vi "SV TDMS Read Scalar (N Ch).vi"(0 "tdms file":refnum<k34>, 1 "offset (0)":i64, 2 "count (-1: all)":i64=-1, 5 "group name in":string, 7 "channel names in":string[](array[string]), 11 "error in":errorcluster) -> (3 "scale labels":T1(array[cluster]), 4 "tdms file out":refnum<k34>, 6 "group name out":string, 8 "channel names out":string[](array[string]), 10 "values":dbl[][](array[numeric]), 13 "scalar function info":T2={"scalar function type"=10, "scalar function subtype"=19, " x-dimension"=0} {"scalar function type" items=["Speed"=3, "Ratio"=6, "Count"=7, "-"=9, "Level"=10, "-"=19, "None"=98]; "scalar function subtype" items=["Value"=19, "DC"=11, "AC"=12, "RMS^2"=13, "RMS"=14, "Peak"=15, "Peak to peak"=16, "-"=20, "Phase"=33, "-"=90, "None"=98, "Unknown"=99]; "x-dimension" items=["Time (s)"=0, "Frequency-CB (Hz)"=1, "Frequency-CPB (Hz)"=1248, "Frequency-Arbitrary (Hz)"=2357, "Quefrency (s)"=2, "Revolutions (rev)"=3, "Order"=4, "Speed (RPM)"=11, "Speed (rad/s)"=21, "Critical Band"=31, "Critical Band Rate (Bark)"=32, "None"=98, "Index"=65535]}, 14 "end of file":bool, 15 "error out":errorcluster)   [LabVIEW 2017]
doc: "Reads the specified .tdms file and returns data in a format specific to the polymorphic instance selected."
uses:
  <vilib>/addons/_NISVFA/_Shared subVIs/Controls/NI Scalar Function Info.ctl
  <vilib>/addons/_NISVFA/_Shared subVIs/Controls/svc_X-Axis Units.ctl
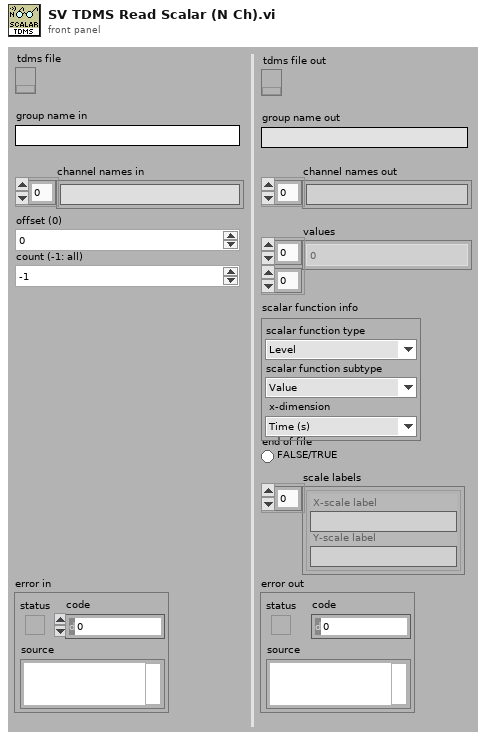
[diagram p1: front panel]
types:
  T1 = cluster{"X-scale label":string, "Y-scale label":string}[]
  T2 = typedef "NI Scalar Function Info.ctl" = cluster{"scalar function type":u16, "scalar function subtype":u16, " x-dimension":T3}
  T3 = typedef "svc_X-Axis Units.ctl" = u16
  T4 = typedef "NI Function Info.ctl" = cluster{"function type":T5, "function subtype":T6, "X-dimension":T3}
  T5 = typedef "NI Function Type.ctl" = u16
  T6 = typedef "NI Function SubType.ctl" = u16
  T7 = cluster{"X-scale label":string, "Y-scale label":string}
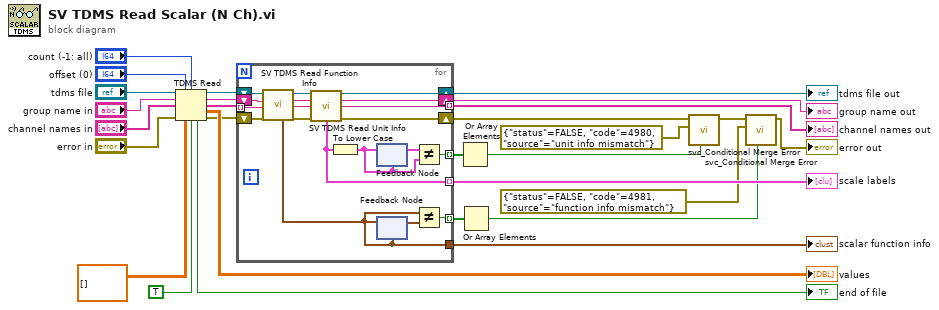
[diagram p0: block diagram]
diagram:
  n1 = TDMS Read(0:"tdms file", 1:"offset (0)", 2:"count (-1: all)", 5:"group name in", 7:"channel names in", 11:"error in", 12:dbl[][] [] ("scaled samples"), 13:TRUE ("return channels in file order? (F)")) -> (4:w17:refnum<k34>, 6:w16:string, 8:w15:string[], 10:→"values":dbl[][], 14:→"end of file":bool, 15:w12:errorcluster)
  n2 = for {
    shift-right: [w47] -> w19
    shift-left: w17 -> [w42]
    shift-right: [w46] -> w18
    shift-left: w16 -> [w41]
    tunnel: w15 -> [w40] mode=indexing
    tunnel: [w45] -> w20 mode=indexing
    shift-right: [w32] -> w7
    shift-left: w12 -> [w36]
    tunnel: [w43] -> w13 mode=indexing
    tunnel: [w33] -> w10
    tunnel: [w31] -> w9 mode=indexing
    tunnel: [w30] -> w8 mode=indexing
    n3 = call <vilib>:"SV TDMS Read Function Info.vi"("error in (no error)"=w36, "channel name"=w40, "group name"=w41, "tdms file in"=w42) -> ("error out"=w37:errorcluster, "channel name out"=w38:string, "group name out"=w39:string, "tdms file out"=w35:refnum<k34>, "function info"=w33:T4)  [unwired: 2 in, 1 out]
    n4 = call <vilib>:"SV TDMS Read Unit Info.vi"("tdms file"=w35, "group name"=w39, "channel name"=w38, "error in (no error)"=w37) -> ("tdms file out"=w47:refnum<k34>, "group name out"=w46:string, "channel name out"=w45:string, "scale labels"=w43:T7, "error out"=w32:errorcluster)  [unwired: 6 in, 1 out]
    n5 = To Lower Case(string=w43) -> (all lower case string=w29:T7)
    n6 = feedback-in #1(w29) -> ()
    n7 = feedback #1(w29) -> (w44:T7)
    n8 = feedback #2(w33) -> (w34:T4)
    n9 = feedback-in #2(w33) -> ()
    n10 = Not Equal?(x=w44, y=w29) -> (x != y?=w31:bool)
    n11 = Not Equal?(x=w33, y=w34) -> (x != y?=w30:bool)
  }
  "channel names out" <- w20
  "group name out" <- w18
  "tdms file out" <- w19
  "scalar function info" <- w10
  "scale labels" <- w13
  n12 = Or Array Elements(Boolean array=w9) -> (logical OR=w6:bool)
  n13 = Or Array Elements(Boolean array=w8) -> (logical OR=w2:bool)
  n14 = call <vilib>:"svc_Conditional Merge Error.vi"("merge"=w6, "new error"=errorcluster {"status"=FALSE, "code"=4980, "source"="unit info mismatch"} ("error out"), "error in (no error)"=w7) -> ("error out"=w4:errorcluster)  [unwired: 8 in]
  n15 = call <vilib>:"svc_Conditional Merge Error.vi"("merge"=w2, "new error"=errorcluster {"status"=FALSE, "code"=4981, "source"="function info mismatch"} ("error out"), "error in (no error)"=w4) -> ("error out"=→"error out":errorcluster)  [unwired: 8 in]
